vi "Step.vi"() -> ()   [LabVIEW 2017]
panel:
  in  "Mover":bool
  out "Actual Position":dbl
  in  "Step":dbl
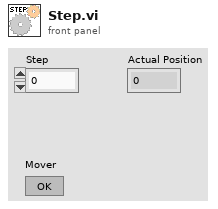
[diagram p1: front panel]
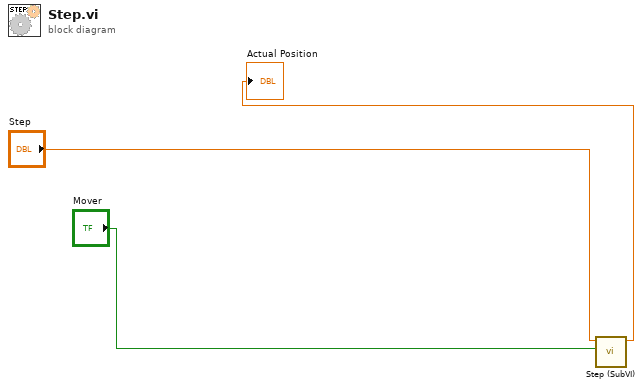
[diagram p0: block diagram]
diagram:
  n1 = call "Step (SubVI).vi"("Mover"="Mover", "Step"="Step") -> ("Numeric"=→"Actual Position":dbl)  [unwired: 9 in]
